vi "Retrieve from DataBase.vi"(8 "error in (no error)":errorcluster, 10 "Search Criteria":string, 11 "DAO in":refnum<class "Object DAO.lvclass">) -> (0 "error out":errorcluster, 3 "DAO out":refnum<class "Object DAO.lvclass">)   [LabVIEW 2020, in "Object DAO.lvclass"]
uses:
  Object DAO.lvclass
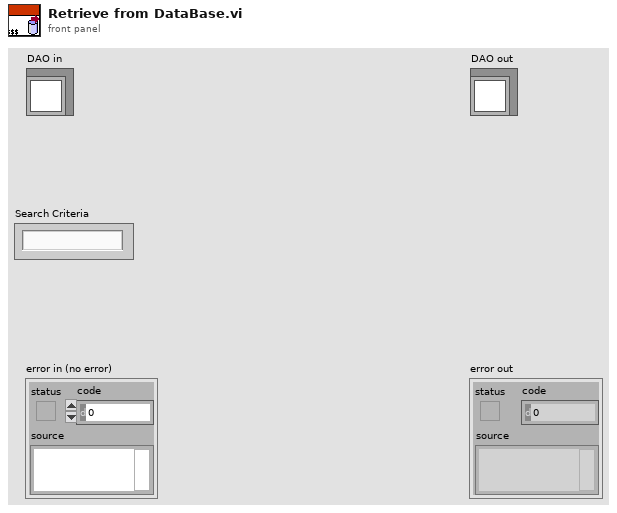
[diagram p1: front panel]
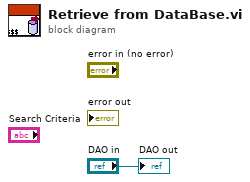
[diagram p0: block diagram]
diagram:
  "DAO out" <- "DAO in"
